vi "Save Data.vi"(9 "Save File":bool, 10 "Waveforms in":waveform(dbl)[](array[waveform]), 11 "deleted path":path) -> ()   [LabVIEW 2021]
uses:
  <vilib>/Waveform/WDTFileIO.llb/Export Waveforms To Spreadsheet File (1D).vi
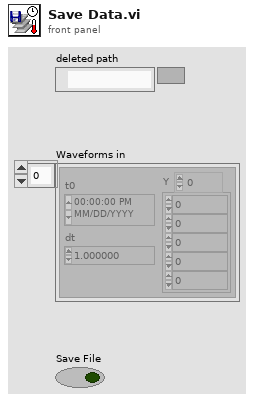
[diagram p1: front panel]
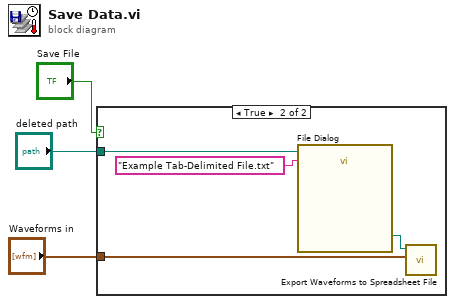
[diagram p0: block diagram]
diagram:
  n1 = case shown="True" "Save File" {
    tunnel: "Waveforms in" -> [_ w7]
    tunnel: "deleted path" -> [_ w4]
    frame False {
    }
    frame True {
      n2 = call "File Dialog"("start path"=w4, "default name"="Example Tab-Delimited File.txt") -> ("selected path"=w5:path)  [unwired: 10 in, 3 out]
      n3 = call-poly <vilib>:"Export Waveforms to Spreadsheet File.vi"("waveforms"=w7, "file path (dialog if empty)"=w5) -> ()  [unwired: 8 in, 2 out]
    }
  }
